vi "Insert View.vi"(8 "error in (no error)":errorcluster, 10 "SubPnl Refnum":refnum<vi>, 11 "MultiSubscriber In":refnum<class "MultiSubscriber.lvclass">) -> (0 "error out":errorcluster, 3 "MultiSubscriber Out":refnum<class "MultiSubscriber.lvclass">)   [LabVIEW 2015, in "TestActors.lvlib" / "MultiSubscriber.lvclass"]
uses:
  MultiSubscriber.lvclass
  MultiSubscriber.lvclass/MultiSubscriber.ctl
  Framework/IViewable/IViewable/IViewable.lvclass
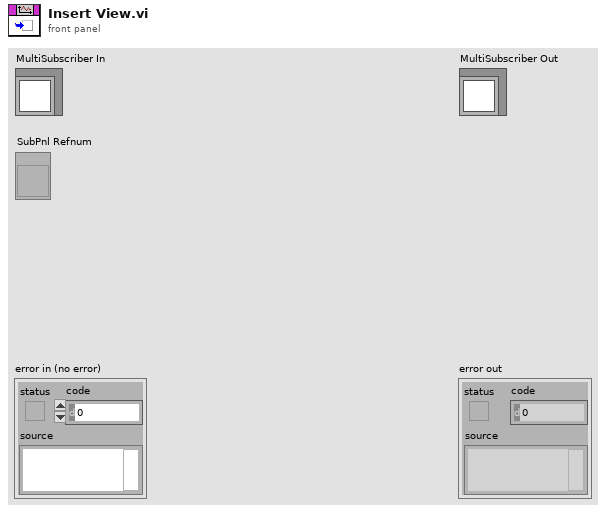
[diagram p1: front panel]
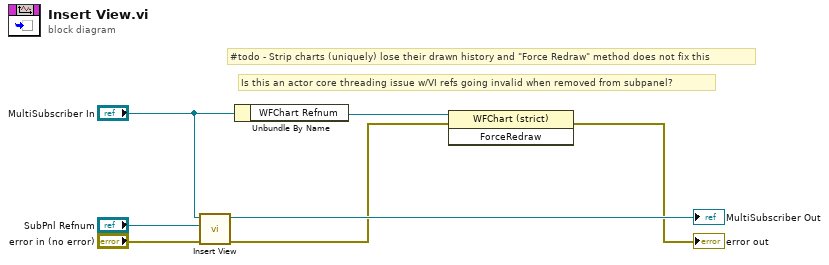
[diagram p0: block diagram]
diagram:
  # "Is this an actor core threading issue w/VI refs going invalid when removed from subpanel?"
  # "#todo - Strip charts (uniquely) lose their drawn history and \"Force Redraw\" method does not fix this"
  n1 = call-parent "Insert View.vi"("error in (no error)"="error in (no error)", "SubPnl Refnum"="SubPnl Refnum", "IViewable in"="MultiSubscriber In") -> ("error out"=w2:errorcluster, "IViewable out"=→"MultiSubscriber Out":refnum<class "MultiSubscriber.lvclass">)  [unwired: 7 in]
  n2 = Unbundle By Name("MultiSubscriber In") -> ("WFChart Refnum"=w3:refnum<vi>)
  n3 = invoke class="WFChart (strict)" method="ForceRedraw"(reference=w3, error in=w2) -> (error out=→"error out":errorcluster)  [unwired: 1 in, 2 out]
